vi "Histogram Main.vi"() -> ()   [LabVIEW 2014]
uses:
  Consumer Message.ctl
  <vilib>/ErrorRing/Error Ring.xnode
panel:
  out "Waveform Chart":dbl[](graph)
  in  "Snapshot":bool
  out "Histogram":cluster{"histogram":dbl[], "x axis":dbl[]}(graph)
  out "Consumer Shutdown?":bool
  in  "Stop":bool
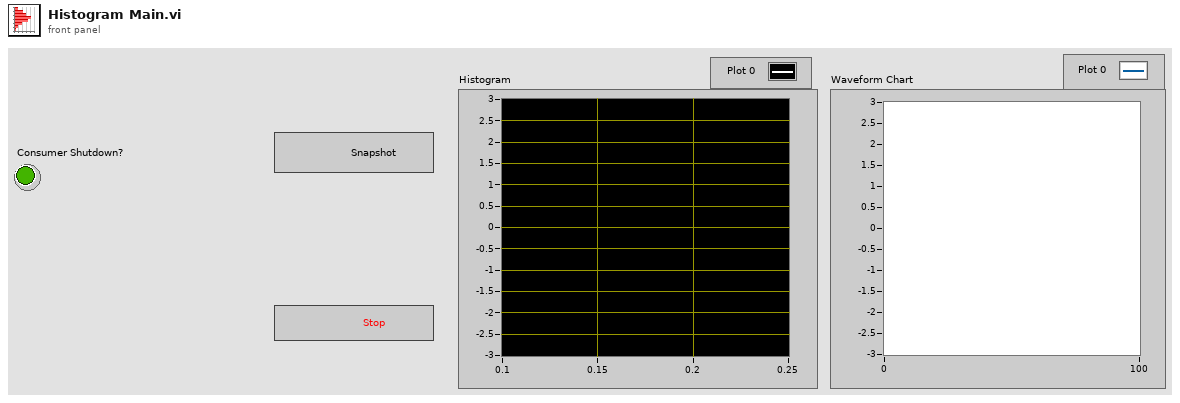
[diagram p1: front panel]
types:
  T1 = typedef "Consumer Message.ctl" = cluster{"Consumer State":string, "Boolean Data":bool, "Numeric Data":i32, "Signal":dbl[], "Error":errorcluster}
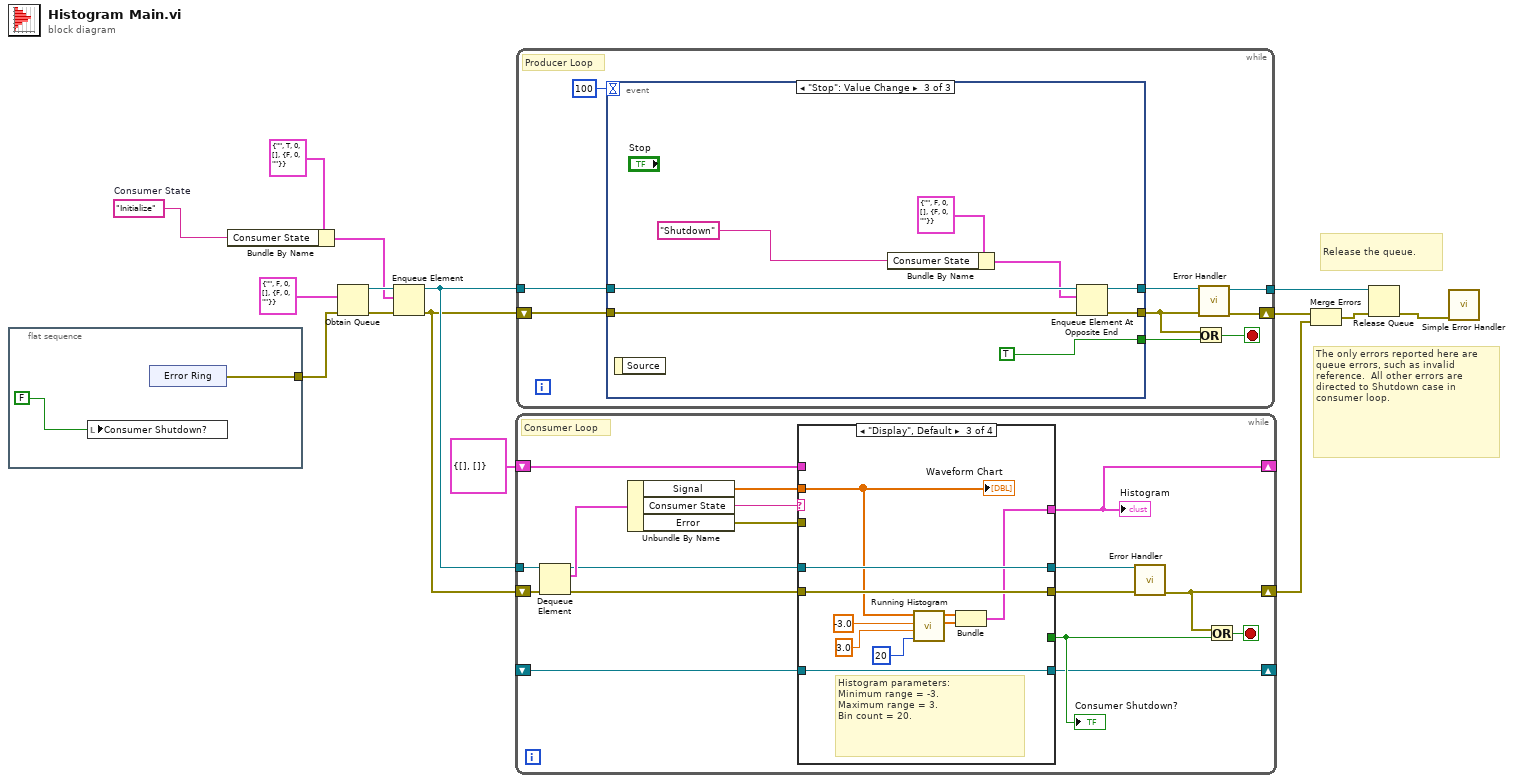
[diagram p0: block diagram]
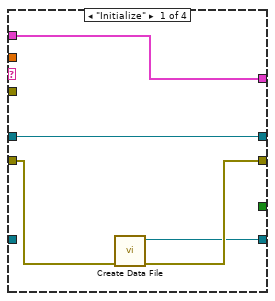
[diagram p2: hidden frame]
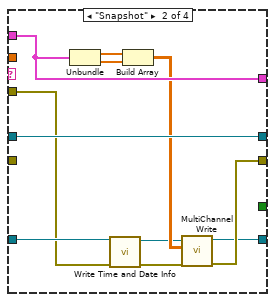
[diagram p3: hidden frame]
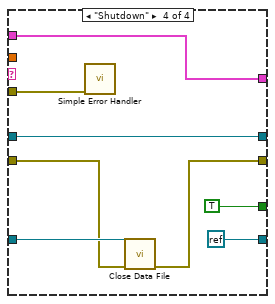
[diagram p4: hidden frame]
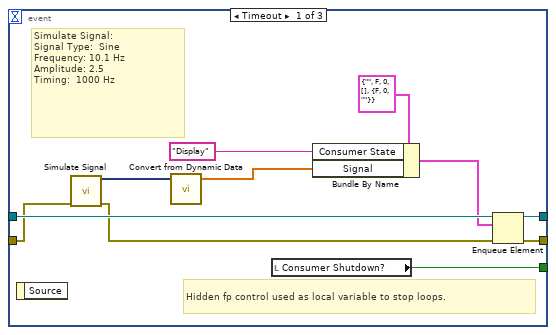
[diagram p5: hidden frame]
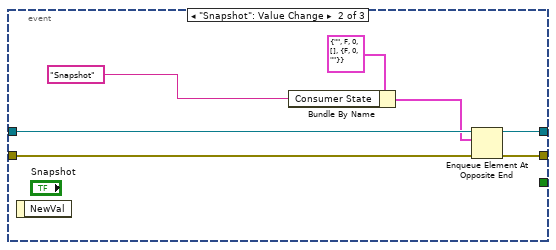
[diagram p6: hidden frame]
diagram:
  w8 = "Initialize"  # Consumer State
  # "Release the queue."
  # "The only errors reported here are queue errors, such as invalid reference.  All other errors are directed to Shutdown case in consumer loop."
  n1 = flat-sequence {
    tunnel: [w16] -> w11
    frame #0 {
      n2 = local write "Consumer Shutdown?"(FALSE ("Stop Loops (local)")) -> ()
      n3 = xnode "Error Ring"() -> ("error out"=w16:errorcluster)
    }
  }
  n4 = Bundle By Name(cluster=T1 {"Consumer State"="", "Boolean Data"=TRUE, "Numeric Data"=0, "Signal"=[], "Error"={"status"=FALSE, "code"=0, "source"=""}} ("Consumer Message"), "Consumer State"=w8) -> (w9:T1)
  n5 = Obtain Queue(element data type=T1 {"Consumer State"="", "Boolean Data"=FALSE, "Numeric Data"=0, "Signal"=[], "Error"={"status"=FALSE, "code"=0, "source"=""}}, error in (no error)=w11) -> (queue out=w13:refnum<queue>, error out=w15:errorcluster)  [unwired: 3 in, 1 out]
  n6 = Enqueue Element(queue=w13, element=w9, error in (no error)=w15) -> (queue out=w12:refnum<queue>, error out=w2:errorcluster)  [unwired: 1 in, 1 out]
  n7 = while {
    tunnel: w12 -> [w35]
    shift-right: [w26] -> w6
    shift-left: w2 -> [w34]
    shift-right: [w19] -> _
    shift-left: cluster{"histogram":dbl[], "x axis":dbl[]} {"histogram"=[], "x axis"=[]} -> [w23]
    shift-right: [w20] -> _
    shift-left: _ -> [w21]
    stop <- w27 stop-if-true
    # "Consumer Loop"
    n8 = Dequeue Element(queue=w35, error in (no error)=w34) -> (queue out=w25:refnum<queue>, element=w33:T1, error out=w24:errorcluster)  [unwired: 1 in, 1 out]
    n9 = Unbundle By Name(w33) -> ("Signal"=w22:dbl[], "Consumer State"=w32:string, "Error"=w29:errorcluster)
    n10 = case shown="\"Display\", Default" w32 {
      tunnel: [_ _ _ TRUE] -> w28
      tunnel: w24 -> [w38 _ w60 w64]
      tunnel: [w37 w47 w60 w63] -> w31
      tunnel: w25 -> [w40 w51 w61 w67]
      tunnel: [w40 w51 w61 w67] -> w30
      tunnel: w29 -> [_ w41 _ w68]
      tunnel: [w39 w49 w57 w66] -> w19
      tunnel: w23 -> [w39 w49 _ w66]
      tunnel: w22 -> [_ _ w55 _]
      tunnel: w21 -> [_ w42 w56 w65]
      tunnel: [w36 w46 w56 refnum<k0> refnum] -> w20
      frame "Initialize" {
        n11 = call "Create Data File.vi"("Error In"=w38) -> ("Error Out"=w37:errorcluster, "File Refnum"=w36:refnum<file>)  [unwired: 9 in]
      }
      frame "Snapshot" {
        n12 = Unbundle(w49) -> ("histogram"=w45:dbl[], "x axis"=w50:dbl[])
        n13 = call "Write Time and Date Info.vi"("Error In"=w41, "File Refnum In"=w42) -> ("Error Out"=w43:errorcluster, "File Refnum Out"=w44:refnum<file>)  [unwired: 6 in]
        n14 = Build Array(w45, w50) -> (w48:dbl[][])
        n15 = call "MultiChannel Write.vi"("Error In"=w43, "Data to Log"=w48, "File Refnum In"=w44) -> ("Error Out"=w47:errorcluster, "File Refnum Out"=w46:refnum<file>)  [unwired: 7 in]
      }
      frame "Display", Default {
        # "Histogram parameters:\nMinimum range = -3.\nMaximum range = 3. \nBin count = 20."
        n16 = call "Running Histogram.vi"("bins"=20, "max"=3.0, "min"=-3.0, "input data"=w55) -> ("x axis"=w58:dbl[], "histogram"=w59:dbl[])  [unwired: 4 in, 2 out]
        n17 = Bundle("histogram"=w59, "x axis"=w58) -> (w57:cluster{"histogram":dbl[], "x axis":dbl[]})  [unwired: 1 in]
        "Waveform Chart" <- w55
      }
      frame "Shutdown" {
        n18 = call <vilib>:"Simple Error Handler.vi"("error in (no error)"=w68) -> ()  [unwired: 4 in, 5 out]
        n19 = call "Close Data File.vi"("error in"=w64, "File Refnum In"=w65) -> ("error out"=w63:errorcluster)  [unwired: 9 in]
      }
    }
    "Consumer Shutdown?" <- w28
    "Histogram" <- w19
    n20 = call "Error Handler.vi"("error in"=w31, "queue in"=w30) -> ("error out"=w26:errorcluster)  [unwired: 8 in, 1 out]
    n21 = Or(x=w26, y=w28) -> (x .or. y?=w27:bool)
  }
  n22 = while {
    tunnel: w12 -> [w78]
    shift-right: [w71] -> w7
    shift-left: w2 -> [w77]
    tunnel: [w70] -> w1
    stop <- w73 stop-if-true
    # "Producer Loop"
    n23 = event shown="[2] \"Stop\": Value Change" {
      selector: _ -> [_ _ _]
      dyn-events: _ -> [_ _ _]
      timeout: 100 -> [_ _ _]
      tunnel: w78 -> [w88 w95 w104]
      tunnel: w77 -> [w81 w94 w102]
      tunnel: [w83 w96 w101] -> w72
      tunnel: [w89 _ TRUE] -> w74
      tunnel: [w84 w91 w100] -> w76
      event Timeout {
        # "Simulate Signal:\nSignal Type:  Sine\nFrequency: 10.1 Hz\nAmplitude: 2.5\nTiming:  1000 Hz"
        # "Hidden fp control used as local variable to stop loops."
        n24 = event-data() -> ()  [unwired: 1 in, 1 out]
        n25 = call "Simulate Signal"("error in (no error)"=w81) -> ("Sine with Uniform Noise"=w79:dynamicdata, "error out"=w80:errorcluster)  [unwired: 13 in]
        n26 = call "Convert from Dynamic Data"("Dynamic Data Type"=w79) -> ("Array"=w82:dbl[])  [unwired: 3 in]
        n27 = local read "Consumer Shutdown?"() -> (w89:bool)
        n28 = Bundle By Name(cluster=T1 {"Consumer State"="", "Boolean Data"=FALSE, "Numeric Data"=0, "Signal"=[], "Error"={"status"=FALSE, "code"=0, "source"=""}}, "Consumer State"="Display", "Signal"=w82) -> (w86:T1)
        n29 = Enqueue Element(queue=w88, element=w86, error in (no error)=w80) -> (queue out=w84:refnum<queue>, error out=w83:errorcluster)  [unwired: 1 in, 1 out]
      }
      event "Snapshot": Value Change {
        n30 = event-data() -> ()  [unwired: 1 in, 1 out]
        n31 = Bundle By Name(cluster=T1 {"Consumer State"="", "Boolean Data"=FALSE, "Numeric Data"=0, "Signal"=[], "Error"={"status"=FALSE, "code"=0, "source"=""}}, "Consumer State"="Snapshot" ("String Data")) -> (w92:T1)
        n32 = Enqueue Element At Opposite End(queue=w95, element=w92, error in (no error)=w94) -> (queue out=w91:refnum<queue>, error out=w96:errorcluster)  [unwired: 1 in, 1 out]
      }
      event "Stop": Value Change {
        n33 = event-data() -> ()  [unwired: 1 in, 1 out]
        n34 = Bundle By Name(cluster=T1 {"Consumer State"="", "Boolean Data"=FALSE, "Numeric Data"=0, "Signal"=[], "Error"={"status"=FALSE, "code"=0, "source"=""}}, "Consumer State"="Shutdown") -> (w97:T1)
        n35 = Enqueue Element At Opposite End(queue=w104, element=w97, error in (no error)=w102) -> (queue out=w100:refnum<queue>, error out=w101:errorcluster)  [unwired: 1 in, 1 out]
      }
    }
    n36 = Or(x=w72, y=w74) -> (x .or. y?=w73:bool)
    n37 = call "Error Handler.vi"("error in"=w72, "queue in"=w76) -> ("error out"=w71:errorcluster, "queue out"=w70:refnum<queue>)  [unwired: 8 in]
  }
  n38 = Merge Errors(w7, w6) -> (w4:errorcluster)
  n39 = Release Queue(queue=w1, error in (no error)=w4) -> (error out=w3:errorcluster)  [unwired: 1 in, 2 out]
  n40 = call <vilib>:"Simple Error Handler.vi"("error in (no error)"=w3) -> ()  [unwired: 4 in, 5 out]
